vi "Close.vi"(8 "error in (no error)":errorcluster, 11 "uService Template in":refnum<class "Run Config Manager.lvclass">) -> (0 "error out":errorcluster, 3 "uService Template out":refnum<class "Run Config Manager.lvclass">)   [LabVIEW 2026, in "TALOS.lvlib" / "Run Config Manager.lvlib" / "Run Config Manager.lvclass"]
uses:
  Run Config Manager.lvclass
  Father of all uServices/Father of all uServices/Father of all uServices.lvclass
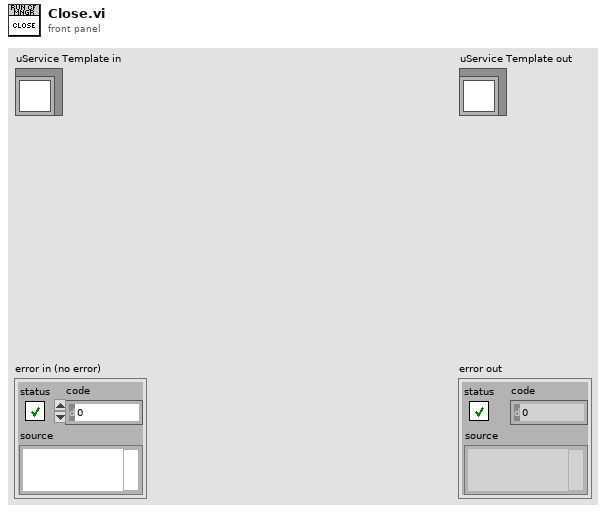
[diagram p1: front panel]
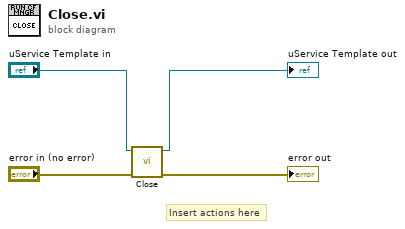
[diagram p0: block diagram]
diagram:
  # "Insert actions here"
  n1 = call-parent "Close.vi"("error in (no error)"="error in (no error)", "uService Template in"="uService Template in") -> ("error out"=→"error out":errorcluster, "uService Template out"=→"uService Template out":refnum<class "Run Config Manager.lvclass">)  [unwired: 8 in]
